vi "Add Points to Series_DBL-DBL-Name.vi"(6 "YValuesPerPoint":i32=1, 8 "error in (no error)":errorcluster, 9 "Data":cluster{"X":dbl, "Y":dbl, "Name":string}[](array[cluster])=[{"X"=0.0, "Y"=0.0, "Name"=""}, {"X"=0.0, "Y"=0.0, "Name"=""}, {"X"=0.0, "Y"=0.0, "Name"=""}, {"X"=0.0, "Y"=0.0, "Name"=""}, {"X"=0.0, "Y"=0.0, "Name"=""}, {"X"=0.0, "Y"=0.0, "Name"=""}, {"X"=0.0, "Y"=0.0, "Name"=""}, {"X"=0.0, "Y"=0.0, "Name"=""}], 10 ".NET MSChart Series":refnum<k24>) -> (0 "error out":errorcluster)   [LabVIEW 2015, in "Graph Extensions MSChart.lvlib"]
uses:
  Graph Extensions MSChart.lvlib
  System.Windows.Forms.DataVisualization
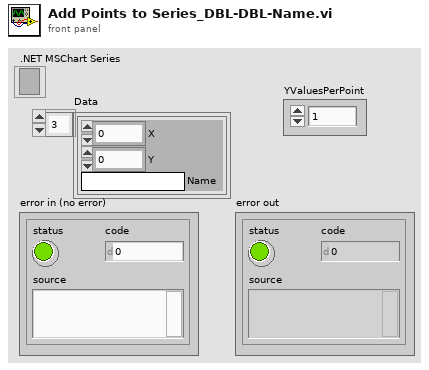
[diagram p1: front panel]
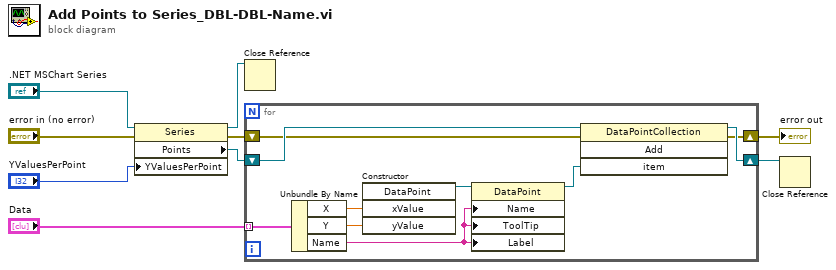
[diagram p0: block diagram]
diagram:
  n1 = property class="Series"(reference=".NET MSChart Series", error in="error in (no error)", "YValuesPerPoint"="YValuesPerPoint") -> (reference out=w6:refnum<k24>, error out=w4:errorcluster, "Points"=w5:refnum<k24>)
  n2 = Close Reference(reference=w6) -> ()  [unwired: 1 in, 1 out]
  n3 = for {
    tunnel: "Data" -> [w16] mode=indexing
    shift-right: [w18] -> w3
    shift-left: w5 -> [w19]
    shift-right: [w10] -> w2
    shift-left: w4 -> [w17]
    n4 = Unbundle By Name(w16) -> ("X"=w15:dbl, "Y"=w14:dbl, "Name"=w12:string)
    n5 = constructor class="DataPoint"("xValue"=w15, "yValue"=w14) -> (reference out=w11:refnum<k24>)  [unwired: 3 in, 4 out]
    n6 = property class="DataPoint"(reference=w11, "Name"=w12, "ToolTip"=w12, "Label"=w12) -> (reference out=w13:refnum<k24>)  [unwired: 1 in, 1 out]
    n7 = invoke class="DataPointCollection" method="Add"(reference=w19, error in=w17, "item"=w13) -> (reference out=w18:refnum<k24>, error out=w10:errorcluster)  [unwired: 1 in, 2 out]
  }
  "error out" <- w2
  n8 = Close Reference(reference=w3) -> ()  [unwired: 1 in, 1 out]
